vi "Write timeouts.vi"(8 "error in (no error)":errorcluster, 10 "timeouts":T1={"conn_timeout"=1000, "reconn_timeout"=3000, "N attempt max"=3, "t_reset_TTL"=120000, "write_timeout"=50, "read_timeout"=500, "period"=100}, 11 "MB Param in":refnum<class "MBTCP Param.lvclass">) -> (0 "error out":errorcluster, 3 "MB Param out":refnum<class "MBTCP Param.lvclass">)   [LabVIEW 2021, in "MBParam.lvlib" / "MBTCP Param.lvclass"]
uses:
  MBTCP Param.lvclass
  Typedefs/timeouts.ctl
  MBTCP Param.lvclass/MBTCP Param.ctl
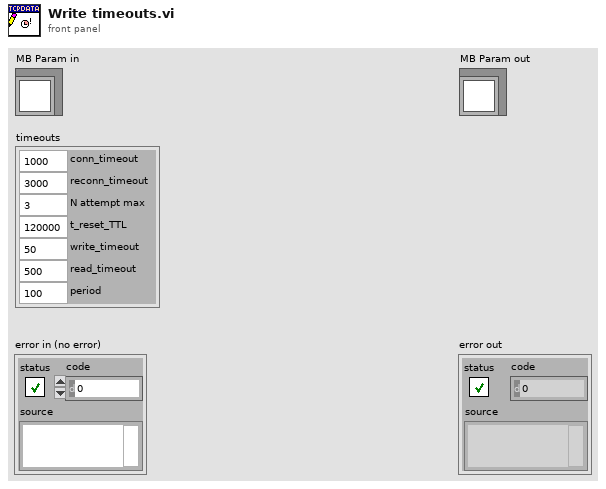
[diagram p1: front panel]
types:
  T1 = typedef "MBParam.lvlib/MBTCP Param.lvclass/timeouts.ctl" = cluster{"conn_timeout":i32, "reconn_timeout":i32, "N attempt max":i32, "t_reset_TTL":i32, "write_timeout":i32, "read_timeout":i32, "period":i32}
  T2 = cluster{"IP address":cluster{"Remote IP Address":string, "Remote Port":u16}, "timeouts":T1}
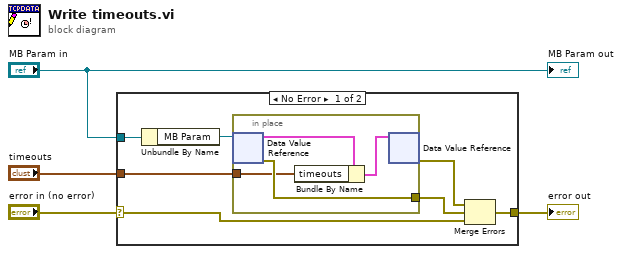
[diagram p0: block diagram]
diagram:
  n1 = case shown="No Error" "error in (no error)" {
    selector: "error in (no error)" -> [w6 w16]
    tunnel: [w10 w16] -> w2
    tunnel: "MB Param in" -> [w11 _]
    tunnel: "timeouts" -> [w5 _]
    frame No Error {
      n2 = Unbundle By Name(w11) -> ("MB Param"=w7:refnum<data-value>)
      n3 = in-place {
        in-place-border: [w15] -> w8
        in-place-border: w5 -> [w13]
        n4 = in-place-dvr #1(w7) -> (w14:T2, w15:errorcluster)
        n5 = Bundle By Name(cluster=w14, "timeouts"=w13) -> (w12:T2)
        n6 = in-place-dvr #1(w12) -> (w9:errorcluster)  [unwired: 1 out]
      }
      n7 = Merge Errors(w9, w8, w6) -> (w10:errorcluster)
    }
    frame Error {
    }
  }
  "error out" <- w2
  "MB Param out" <- "MB Param in"
